vi "CRYWindow Send To SUB VI.vi"(9 "nData":i32, 10 "tFrame_Out":T2, 11 "sAction":string) -> (0 "bResult":bool=TRUE)   [LabVIEW 2013]
uses:
  <vilib>/Utility/miscctls.llb/LVRectTypeDef.ctl
  DataView/VIEW/CRYView Global.vi
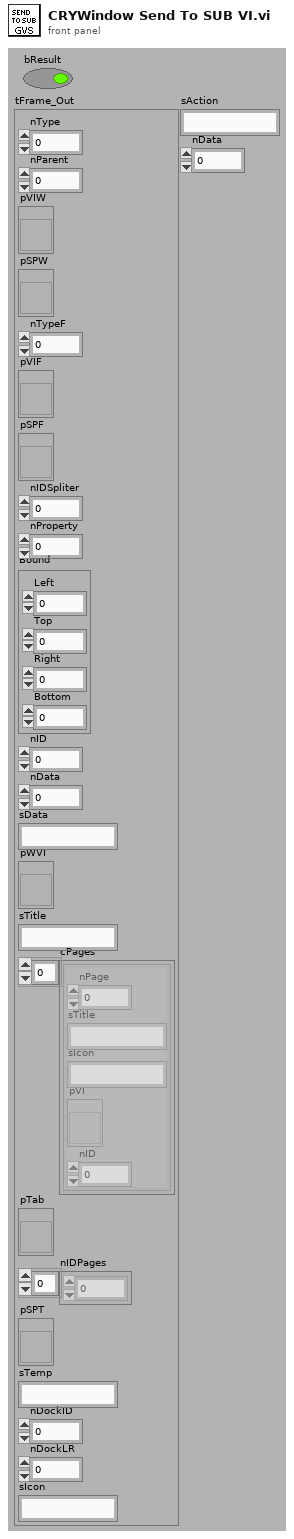
[diagram p1: front panel]
types:
  T1 = typedef "LVRectTypeDef.ctl" = cluster{"Left":i16, "Top":i16, "Right":i16, "Bottom":i16}
  T2 = cluster{"nType":i32, "nParent":i32, "pVIW":refnum<vi>, "pSPW":refnum<vi>, "nTypeF":i32, "pVIF":refnum<vi>, "pSPF":refnum<vi>, "nIDSpliter":i32, "nProperty":i32, "Bound":T1, "nID":i32, "nData":i32, "sData":string, "pWVI":refnum<vi>, "sTitle":string, "cPages":cluster{"nPage":i32, "sTitle":string, "sIcon":string, "pVI":refnum<vi>, "nID":i32}[], "pTab":refnum<vi>, "nIDPages":i32[], "pSPT":refnum<vi>, "sTemp":string, "nDockID":i32, "nDockLR":i32, "sIcon":string}
  T3 = cluster{"sCmdType":string, "nIDView":i32, "sAction":string, "sData":string, "sOption":string, "nData":i32, "nOption":i32, "pVIRef":refnum<vi>, "pSPRef":refnum<vi>, "bWaitRef":refnum<vi>, "Result":variant}
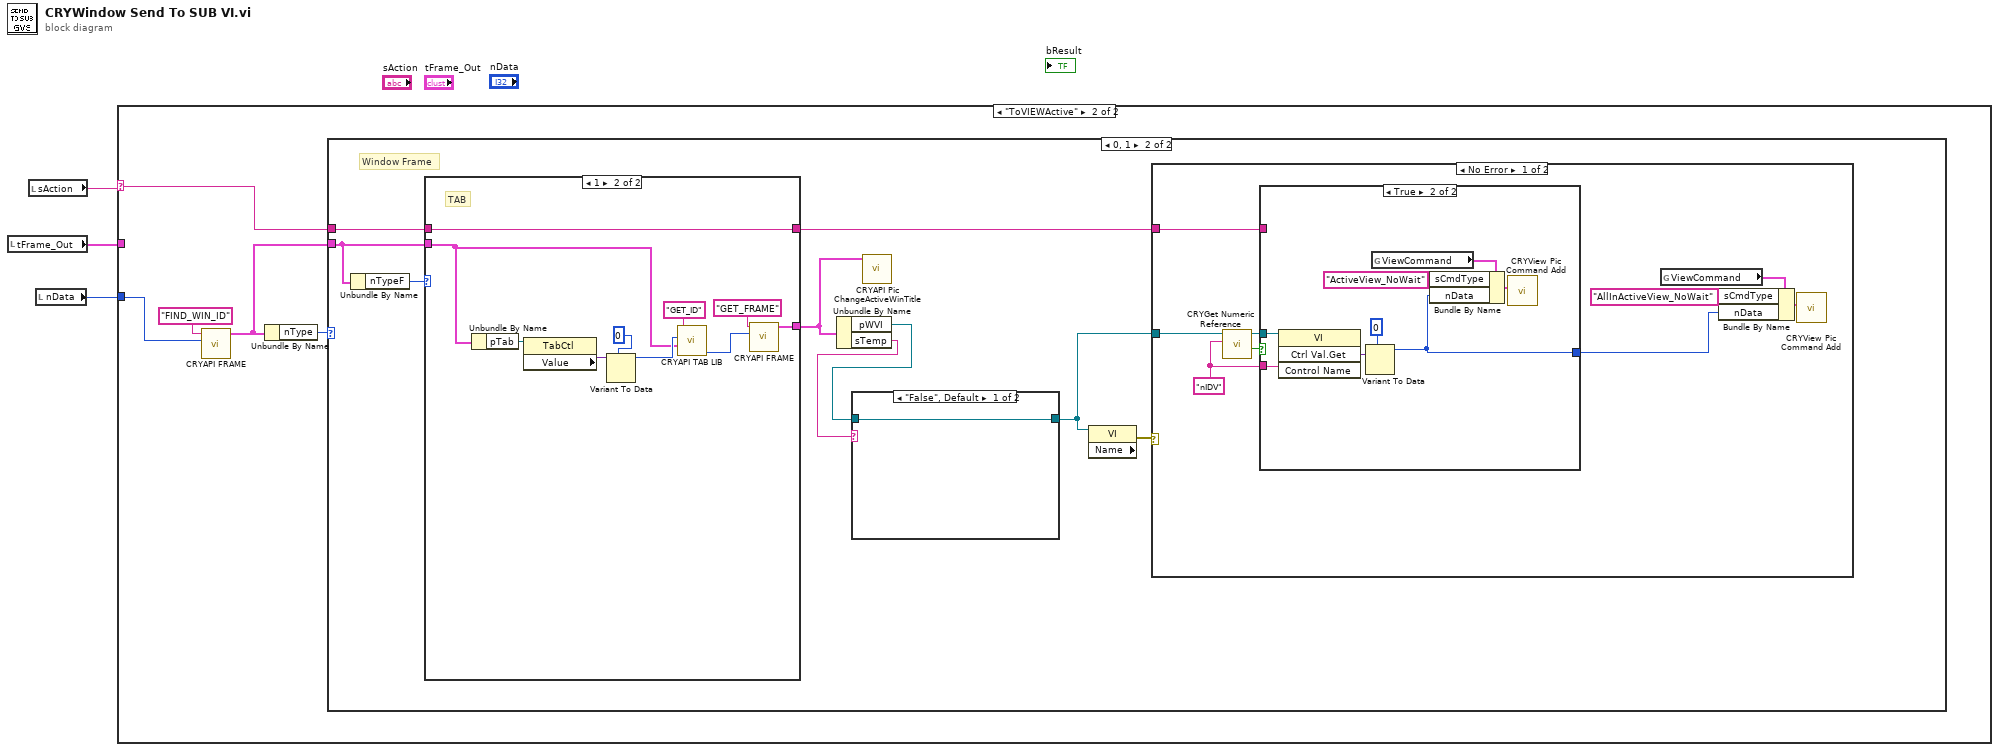
[diagram p0: block diagram]
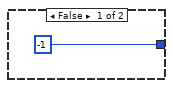
[diagram p4: hidden frame]
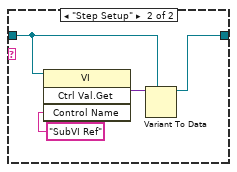
[diagram p6: hidden frame]
diagram:
  n1 = local read "tFrame_Out"() -> (w2:T2)
  n2 = local read "sAction"() -> (w3:string)
  n3 = local read "nData"() -> (w1:i32)
  n4 = case shown="\"ToVIEWActive\"" w3 {
    selector: w3 -> [_ w8]
    tunnel: w2 -> [_ _]
    tunnel: w1 -> [_ w6]
    frame Default {
    }
    frame "ToVIEWActive" {
      n5 = call "CRYAPI FRAME.vi"("nData"=w6, "sAction"="FIND_WIN_ID") -> ("tFrame_Out"=w4:T2)  [unwired: 6 in, 3 out]
      n6 = Unbundle By Name(w4) -> ("nType"=w5:i32)
      n7 = case shown="0, 1" w5 {
        tunnel: w8 -> [_ w16]
        tunnel: w4 -> [_ w15]
        frame Default {
        }
        frame 0, 1 {
          # "Window Frame"
          n8 = Unbundle By Name(w15) -> ("nTypeF"=w17:i32)
          n9 = case shown="1" w17 {
            tunnel: w15 -> [w42 w46]
            tunnel: w16 -> [w41 w43]
            tunnel: [w42 w44] -> w9
            tunnel: [w41 w43] -> w12
            frame Default {
              # "WIN"
            }
            frame 1 {
              # "TAB"
              n10 = Unbundle By Name(w46) -> ("pTab"=w51:refnum<vi>)
              n11 = property class="TabCtl"(reference=w51) -> ("Value"=w50:variant)  [unwired: 1 in, 2 out]
              n12 = Variant To Data(type=0, Variant=w50) -> (data=w47:i32)  [unwired: 1 in, 1 out]
              n13 = call "CRYAPI TAB LIB.vi"("tFrame"=w46, "nData"=w47, "sAction"="GET_ID") -> ("nData_Out"=w45:i32)  [unwired: 6 in, 2 out]
              n14 = call "CRYAPI FRAME.vi"("nData"=w45, "sAction"="GET_FRAME") -> ("tFrame_Out"=w44:T2)  [unwired: 4 in, 5 out]
            }
          }
          n15 = Unbundle By Name(w9) -> ("pWVI"=w13:refnum<vi>, "sTemp"=w14:string)
          n16 = case shown="\"False\", Default" w14 {
            tunnel: w13 -> [w36 w38]
            tunnel: [w36 w37] -> w11
            frame "False", Default {
            }
            frame "Step Setup" {
              n17 = invoke class="VI" method="Ctrl Val.Get"(reference=w38, "Control Name"="SubVI Ref" ("Label Name")) -> ("Get Control Value Variant"=w39:variant)  [unwired: 2 in, 3 out]
              n18 = Variant To Data(type=w38, Variant=w39) -> (data=w37:refnum<vi>)  [unwired: 1 in, 1 out]
            }
          }
          n19 = call "CRYAPI Pic ChangeActiveWinTitle.vi"("tFrame"=w9) -> ()  [unwired: 11 in]
          n20 = property class="VI" props=["Name"](reference=w11) -> (error out=w10:errorcluster)  [unwired: 1 in, 2 out]
          n21 = case shown="No Error" w10 {
            tunnel: w11 -> [w23 _]
            tunnel: w12 -> [w22 _]
            frame No Error {
              w26 = "nIDV" ("Label Name")
              n22 = call "CRYGet Numeric Reference.vi"("Label Name"=w26, "VI Refnum"=w23) -> ("Boolean"=w24:bool, "VI Refnum Out"=w25:refnum<vi>)  [unwired: 7 in, 1 out]
              n23 = case shown="True" w24 {
                tunnel: w25 -> [_ w35]
                tunnel: w26 -> [_ w34]
                tunnel: w22 -> [_ _]
                tunnel: [-1 ("nData_Out") w28] -> w18
                frame False {
                }
                frame True {
                  n24 = invoke class="VI" method="Ctrl Val.Get"(reference=w35, "Control Name"=w34) -> ("Get Control Value Variant"=w33:variant)  [unwired: 2 in, 3 out]
                  n25 = Variant To Data(type=0, Variant=w33) -> (data=w28:i32)  [unwired: 1 in, 1 out]
                  n26 = global read "CRYView Global.vi" "ViewCommand"() -> (w29:T3)
                  n27 = Bundle By Name(cluster=w29, "sCmdType"="ActiveView_NoWait", "nData"=w28) -> (w30:T3)
                  n28 = call "CRYView Pic Command Add.vi"("cCommand"=w30) -> ()  [unwired: 11 in]
                }
              }
              n29 = global read "CRYView Global.vi" "ViewCommand"() -> (w21:T3)
              n30 = Bundle By Name(cluster=w21, "sCmdType"="AllInActiveView_NoWait", "nData"=w18) -> (w20:T3)
              n31 = call "CRYView Pic Command Add.vi"("cCommand"=w20) -> ()  [unwired: 11 in]
            }
            frame Error {
            }
          }
        }
      }
    }
  }
